vi "SetDesiredVoltage(V).vi"(0 "object in":refnum<class "InstrumentBase.lvclass">, 1 "DesiredVoltage(V)":dbl, 5 "error in (no error)":errorcluster) -> (14 "object out":refnum<class "InstrumentBase.lvclass">, 19 "error out":errorcluster)   [LabVIEW 2023, in "InstrumentBase.lvclass"]
uses:
  InstrumentBase.lvclass
  InstrumentBase.lvclass/InstrumentBase.ctl
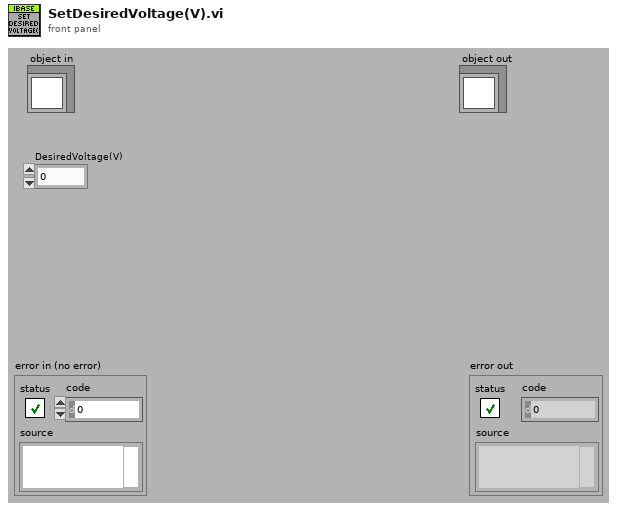
[diagram p1: front panel]
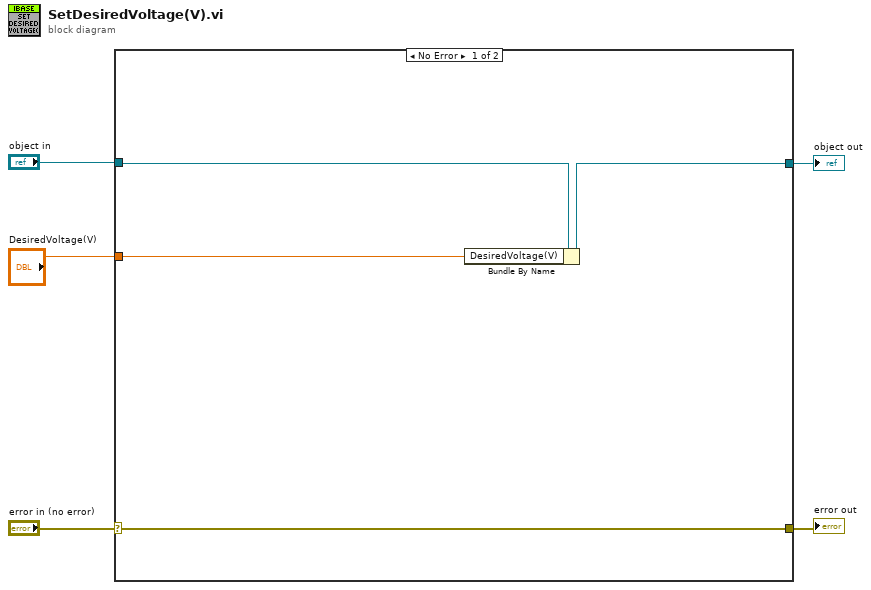
[diagram p0: block diagram]
diagram:
  n1 = case shown="No Error" "error in (no error)" {
    selector: "error in (no error)" -> [w8 w11]
    tunnel: [w8 w11] -> w4
    tunnel: [w6 w10] -> w2
    tunnel: "object in" -> [w7 w10]
    tunnel: "DesiredVoltage(V)" -> [w9 _]
    frame No Error {
      n2 = Bundle By Name(cluster=w7, "DesiredVoltage(V)"=w9) -> (w6:refnum<class "InstrumentBase.lvclass">)
    }
    frame Error {
    }
  }
  "error out" <- w4
  "object out" <- w2
